vi "AddTopic.vi"(8 "error in (no error)":errorcluster, 9 "Topic Actor Descriptor":refnum<class "Topic Actor Descriptor.lvclass">, 10 "Topic Name":string, 11 "Message Broker in":refnum<class "Message Broker.lvclass">) -> (0 "error out":errorcluster, 1 "Transport":refnum<class "Message Transport Queue.lvclass">, 2 "Locked?":bool, 3 "Message Broker out":refnum<class "Message Broker.lvclass">)   [LabVIEW 2016, in "Stream Mediator.lvlib" / "Message Broker.lvclass"]
doc: "--\nCopyright © 2017 Composed SystemsI All rights reserved.\n\nAuthor: Jon McBee <jon.mcbee@composed.io>\n\nThis library is provided \"AS IS\" ,WITHOUT WARRANTIES OR\nCONDITIONS OF ANY KIND, either express or implied.\n\nComposed Systems -- composed.io\n\nStream 0.0.1.1\nJon McBee - Composed Systems\nCopyright (c) 2017, Composed Systems"
uses:
  <userlib>/Composed Systems/Stream/Mediator/Classes/Message Broker/Message Broker.lvclass
  <userlib>/Composed Systems/Stream/Mediator/Classes/Topic Actor Descriptor/Topic Actor Descriptor.lvclass
  <userlib>/Composed Systems/Stream/Mediator/Classes/Message Transport Queue/Message Transport Queue.lvclass
  <userlib>/Composed Systems/Stream/Mediator/Classes/Message Broker/Message Broker.lvclass/Message Broker.ctl
  <userlib>/Composed Systems/Stream/Mediator/Classes/Topic Actor Look Up Table/Topic Actor Look Up Table.lvclass
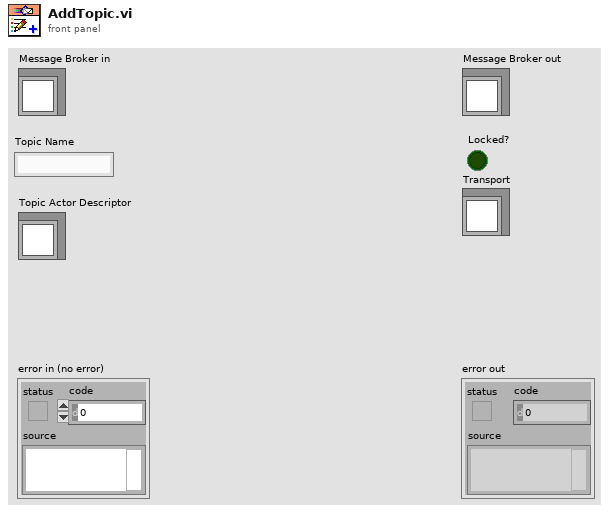
[diagram p1: front panel]
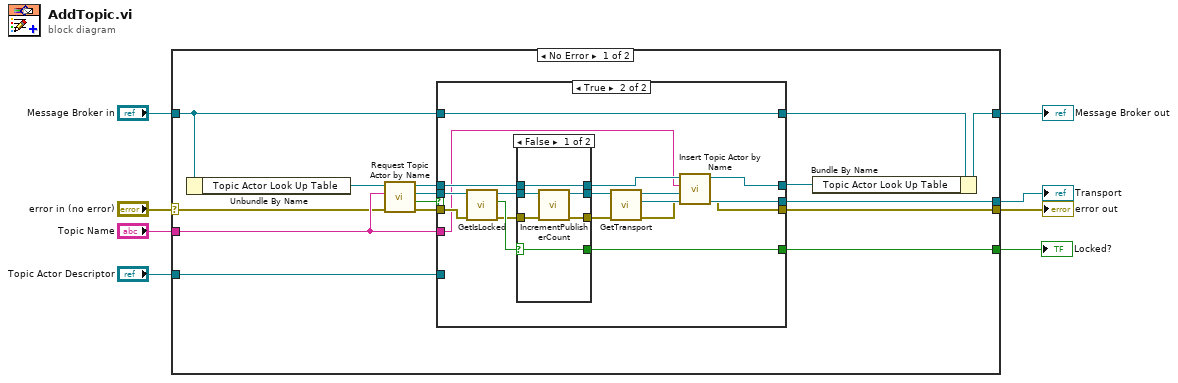
[diagram p0: block diagram]
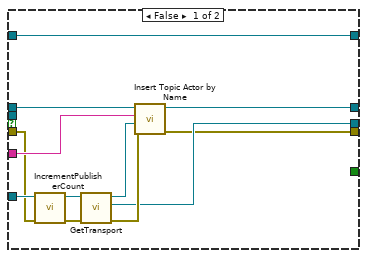
[diagram p2: hidden frame]
diagram:
  n1 = case shown="No Error" "error in (no error)" {
    selector: "error in (no error)" -> [w10 w64]
    tunnel: [w9 w64] -> w7
    tunnel: [w13 w63] -> w5
    tunnel: "Message Broker in" -> [w16 w63]
    tunnel: "Topic Actor Descriptor" -> [w18 _]
    tunnel: "Topic Name" -> [w19 _]
    tunnel: [w15 _] -> w2
    tunnel: [w11 _] -> w1
    frame No Error {
      n2 = Unbundle By Name(w16) -> ("Topic Actor Look Up Table"=w23:refnum<class "Topic Actor Look Up Table.lvclass">)
      n3 = call <userlib>:"Request Topic Actor by Name.vi"("error in (no error)"=w10, "Topic Actor"=w19, "Topic Actor Look Up Table in"=w23) -> ("error out"=w17:errorcluster, "Found?"=w22:bool, "Topic Actor Descriptor"=w20:refnum<class "Topic Actor Descriptor.lvclass">, "Topic Actor Look Up Table out"=w21:refnum<class "Topic Actor Look Up Table.lvclass">)  [unwired: 5 in]
      n4 = case shown="True" w22 {
        tunnel: w21 -> [w35 w43]
        tunnel: w20 -> [_ w52]
        tunnel: w19 -> [w34 w40]
        tunnel: w18 -> [w33 _]
        tunnel: w17 -> [w28 w51]
        tunnel: [w32 w50] -> w14
        tunnel: w16 -> [w32 w50]
        tunnel: [_ w46] -> w15
        tunnel: [w26 w41] -> w12
        tunnel: [w25 w39] -> w11
        tunnel: [w24 w36] -> w9
        frame False {
          n5 = call <userlib>:"IncrementPublisherCount.vi"("error in (no error)"=w28, "Topic Actor Descriptor in"=w33) -> ("error out"=w29:errorcluster, "Topic Actor Descriptor out"=w31:refnum<class "Topic Actor Descriptor.lvclass">)  [unwired: 8 in]
          n6 = call <userlib>:"GetTransport.vi"("error in (no error)"=w29, "Topic Actor Descriptor in"=w31) -> ("error out"=w27:errorcluster, "Transport"=w25:refnum<class "Message Transport Queue.lvclass">, "Topic Actor Descriptor out"=w30:refnum<class "Topic Actor Descriptor.lvclass">)  [unwired: 7 in]
          n7 = call <userlib>:"Insert Topic Actor by Name.vi"("error in (no error)"=w27, "Topic Actor Descriptor"=w30, "Topic Actor"=w34, "Topic Actor Look Up Table in"=w35) -> ("error out"=w24:errorcluster, "Topic Actor Look Up Table out"=w26:refnum<class "Topic Actor Look Up Table.lvclass">)  [unwired: 5 in, 1 out]
        }
        frame True {
          n8 = call <userlib>:"GetIsLocked.vi"("error in (no error)"=w51, "Topic Actor Descriptor in"=w52) -> ("error out"=w47:errorcluster, "Locked?"=w49:bool, "Topic Actor Descriptor out"=w48:refnum<class "Topic Actor Descriptor.lvclass">)  [unwired: 7 in]
          n9 = case shown="False" w49 {
            selector: w49 -> [w54 w60]
            tunnel: w48 -> [w58 w61]
            tunnel: w47 -> [w57 w62]
            tunnel: [w56 w61] -> w45
            tunnel: [w55 w62] -> w44
            tunnel: [w54 w60] -> w46
            tunnel: w43 -> [w53 w59]
            tunnel: [w53 w59] -> w42
            frame False {
              n10 = call <userlib>:"IncrementPublisherCount.vi"("error in (no error)"=w57, "Topic Actor Descriptor in"=w58) -> ("error out"=w55:errorcluster, "Topic Actor Descriptor out"=w56:refnum<class "Topic Actor Descriptor.lvclass">)  [unwired: 8 in]
            }
            frame True {
            }
          }
          n11 = call <userlib>:"GetTransport.vi"("error in (no error)"=w44, "Topic Actor Descriptor in"=w45) -> ("error out"=w37:errorcluster, "Transport"=w39:refnum<class "Message Transport Queue.lvclass">, "Topic Actor Descriptor out"=w38:refnum<class "Topic Actor Descriptor.lvclass">)  [unwired: 7 in]
          n12 = call <userlib>:"Insert Topic Actor by Name.vi"("error in (no error)"=w37, "Topic Actor Descriptor"=w38, "Topic Actor"=w40, "Topic Actor Look Up Table in"=w42) -> ("error out"=w36:errorcluster, "Topic Actor Look Up Table out"=w41:refnum<class "Topic Actor Look Up Table.lvclass">)  [unwired: 5 in, 1 out]
        }
      }
      n13 = Bundle By Name(cluster=w14, "Topic Actor Look Up Table"=w12) -> (w13:refnum<class "Message Broker.lvclass">)
    }
    frame Error {
    }
  }
  "error out" <- w7
  "Message Broker out" <- w5
  "Locked?" <- w2
  "Transport" <- w1
